vi "Add SubPanel to Map.vi"(8 "error in (no error)":errorcluster, 9 "SubPanel Data":T1, 10 "SubPanel Name":string, 11 "CIF_UI in":refnum<class "CIF_UI.lvclass">) -> (0 "error out":errorcluster, 3 "CIF_UI out":refnum<class "CIF_UI.lvclass">)   [LabVIEW 2021, in "CIF_UI.lvclass"]
uses:
  CIF_UI.lvclass
  Typedef/Subpanel Data.ctl
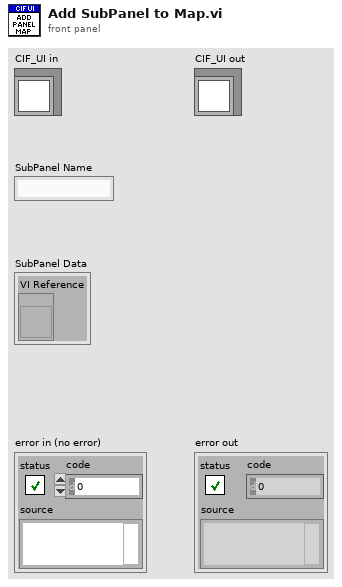
[diagram p1: front panel]
types:
  T1 = typedef "CIF_UI.lvclass/Subpanel Data.ctl" = cluster{"VI Reference":refnum<vi>}
  T2 = typedef "CIF_UI.lvclass/Subpanel Map.ctl" = map{T3, T1}
  T3 = typedef "CIF_UI.lvclass/Subpanel Type.ctl" = enum16{"System", "Errors", "Channel", "Plugin"}
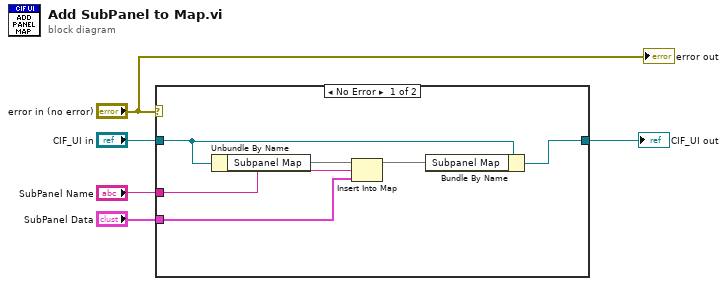
[diagram p0: block diagram]
diagram:
  n1 = case shown="No Error" "error in (no error)" {
    tunnel: [w8 w12] -> w4
    tunnel: "CIF_UI in" -> [w10 w12]
    tunnel: "SubPanel Name" -> [w6 _]
    tunnel: "SubPanel Data" -> [w7 _]
    frame No Error {
      n2 = Unbundle By Name(w10) -> ("Subpanel Map"=w11:T2)
      n3 = Insert Into Map(map in=w11, key=w6, value=w7) -> (map out=w9:T2)  [unwired: 2 out]
      n4 = Bundle By Name(cluster=w10, "Subpanel Map"=w9) -> (w8:refnum<class "CIF_UI.lvclass">)
    }
    frame Error {
    }
  }
  "CIF_UI out" <- w4
  "error out" <- "error in (no error)"
